vi "0037-Sub_map.vi"(7 "error out":errorcluster, 9 "アドレス":i32, 10 "device":T2) -> (0 "error out 2":errorcluster caption="error out", 1 "x = y?":bool, 3 "device 2":T2)   [LabVIEW 2014]
uses:
  <userlib>/LV-CP2112_2014/LVProject/private/CP2112_device.ctl
  <userlib>/LV-CP2112_2014/LVProject/private/CP2112_SMBUS_S0.ctl
panel:
  out "HID_SMBUS_S0":T1
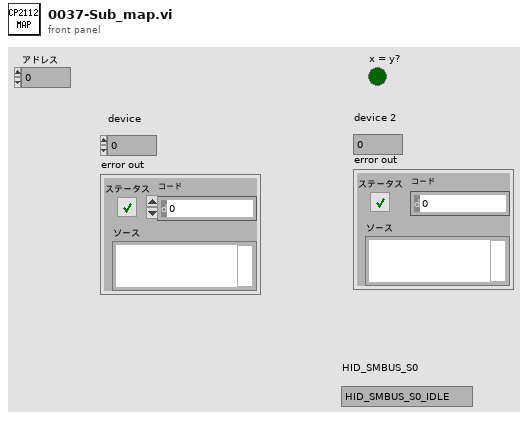
[diagram p1: front panel]
types:
  T1 = typedef "CP2112_SMBUS_S0.ctl" = enum8{"HID_SMBUS_S0_IDLE", "HID_SMBUS_S0_BUSY", "HID_SMBUS_S0_COMPLETE", "HID_SMBUS_S0_ERROR"}
  T2 = typedef "CP2112_device.ctl" = i32
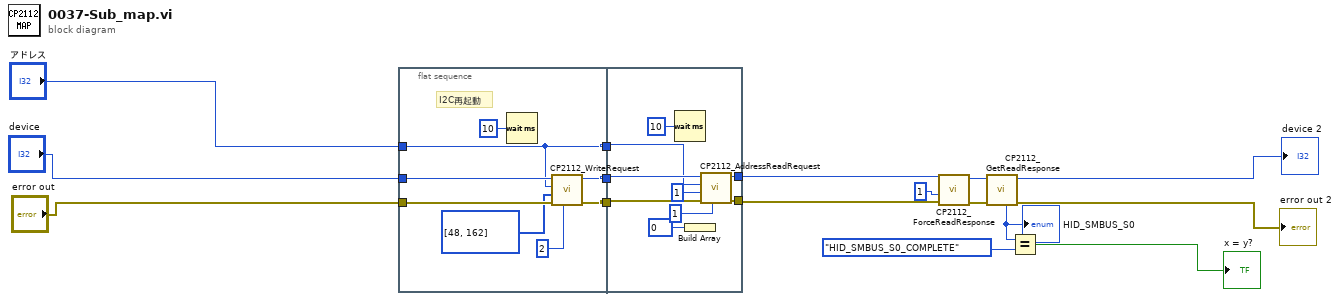
[diagram p0: block diagram]
diagram:
  n1 = flat-sequence {
    tunnel: "device" -> [w24]
    tunnel: "error out" -> [w22]
    tunnel: "アドレス" -> [w20]
    tunnel: [w23] -> w10
    tunnel: [w21] -> w9
    tunnel: [w20] -> w8
    tunnel: w10 -> [w29]
    tunnel: w9 -> [w30]
    tunnel: w8 -> [w28]
    tunnel: [w26] -> w7
    tunnel: [w25] -> w6
    frame #0 {
      # "I2C再起動"
      n2 = Wait (ms)(milliseconds to wait=u32 10 ("ミリ秒待機時間")) -> ()  [unwired: 1 out]
      n3 = call <userlib>:"CP2112_WriteRequest.vi"("numBytesToWrite"=u8 2, "error in (no error)"=w22, "buffer"=u8[] [48, 162], "slaveAddress"=w20, "device"=w24) -> ("error out"=w21:errorcluster, "deviceOut"=w23:T2)  [unwired: 4 in, 1 out]
    }
    frame #1 {
      n4 = Wait (ms)(milliseconds to wait=u32 10 ("ミリ秒待機時間")) -> ()  [unwired: 1 out]
      n5 = Build Array(u8 0 ("targetAddressSize")) -> ()  [unwired: 1 out]
      n6 = call <userlib>:"CP2112_AddressReadRequest.vi"("targetAddressSize"=u8 1, "error in (no error)"=w30, "numByteToRead"=i16 1, "slaveAddress"=w28, "device"=w29) -> ("error out"=w26:errorcluster, "deviceOut"=w25:T2)  [unwired: 4 in, 1 out]
    }
  }
  n7 = call <userlib>:"CP2112_ForceReadResponse.vi"("error in (no error)"=w7, "numByteToRead"=i16 1, "device"=w6) -> ("error out"=w16:errorcluster, "deviceOut"=w15:T2)  [unwired: 6 in, 1 out]
  n8 = call <userlib>:"CP2112_GetReadResponse.vi"("error in (no error)"=w16, "device"=w15) -> ("error out"=→"error out 2":errorcluster, "deviceOut"=→"device 2":T2, "HID_SMBUS_S0"=w12:T1)  [unwired: 4 in, 3 out]
  "HID_SMBUS_S0" <- w12
  n9 = Equal?(x=w12, y=CP2112_SMBUS_S0."HID_SMBUS_S0_COMPLETE" ("HID_SMBUS_S0")) -> (x = y?=→"x = y?":bool)
